vi "AIT 429 Parameter Page.vi"(8 "error in (no error)":errorcluster, 11 "Node Ptr":T3 format="%.0x") -> (0 "error out":errorcluster)   [LabVIEW 2011, in "AIT 429 Custom Device.lvlib"]
uses:
  AIT 429 Custom Device.lvlib
  <vilib>/NI Veristand/Custom Device API/Custom Device Item Ref.ctl
  Controls and Global/Start Bit.ctl
  Controls and Global/Number of Bits.ctl
  Controls and Global/Global.vi
  <vilib>/NI Veristand/Custom Device API/Get Item Property (U32).vi
  <vilib>/NI Veristand/Custom Device API/Get Item Property (Boolean).vi
  <vilib>/NI Veristand/Custom Device API/Get Item Property (Double).vi
  <vilib>/NI Veristand/Custom Device API/Get Item Property (I32).vi
  <vilib>/NI Veristand/Custom Device API/Set Item Property (I32).vi
  <vilib>/NI Veristand/Custom Device API/Set Item Property (Boolean).vi
  <vilib>/NI Veristand/Custom Device API/Set Item Property (Double).vi
  <vilib>/NI Veristand/Custom Device API/Custom Device API.lvlib
panel:
  out "TiggerDValChange":bool
  in  "Scale Offset":dbl format="%#_6f"
  in  "Scale Factor":dbl format="%#_6f"
  in  "Signed?":bool
  out "Default Value":dbl
  in  "Number of Bits":T1=1 min=1 max=32
  in  "Start Bit":T2=1
  in  "Header":cluster{"Section Name":string}={"Section Name"="AIT 429 Parameter"}
  in  "Description":string
  in  "Name":string
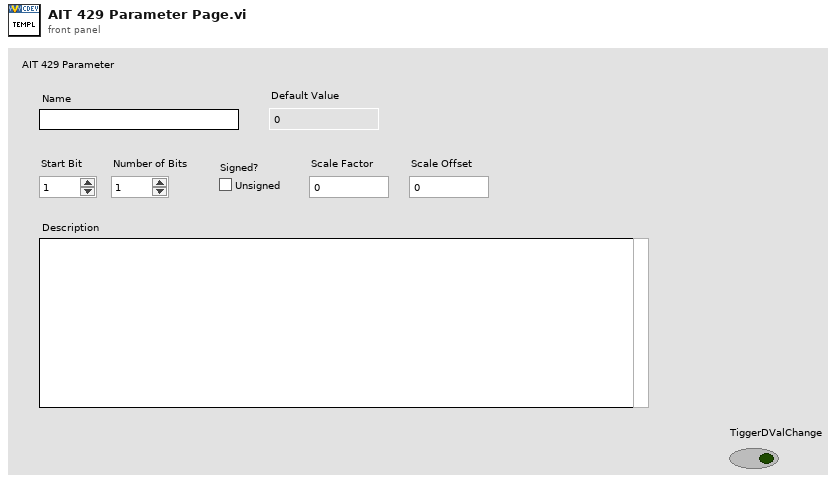
[diagram p1: front panel]
types:
  T1 = typedef "AIT 429 Custom Device.lvlib/Number of Bits.ctl" = i32
  T2 = typedef "AIT 429 Custom Device.lvlib/Start Bit.ctl" = i32
  T3 = typedef "Custom Device API.lvlib/Custom Device Item Ref.ctl" = u64
  T4 = typedef "Custom Device API.lvlib/Custom Device Item Info.ctl" = cluster{"Name":string, "Is Channel":bool, "GUID":string}
  T5 = typedef "Custom Device API.lvlib/Custom Device Channel.ctl" = cluster{"Type":T6, "Units":string, "Default Value":dbl, "Faultable":bool, "Scalable":bool}
  T6 = typedef "Custom Device API.lvlib/Custom Device Channel Type.ctl" = enum16{"Input", "Output"}
  T7 = typedef "Custom Device API.lvlib/Custom Device Commands.ctl" = enum16{"Default", "Item renamed", "Shutdown", "Dynamic button pressed"}
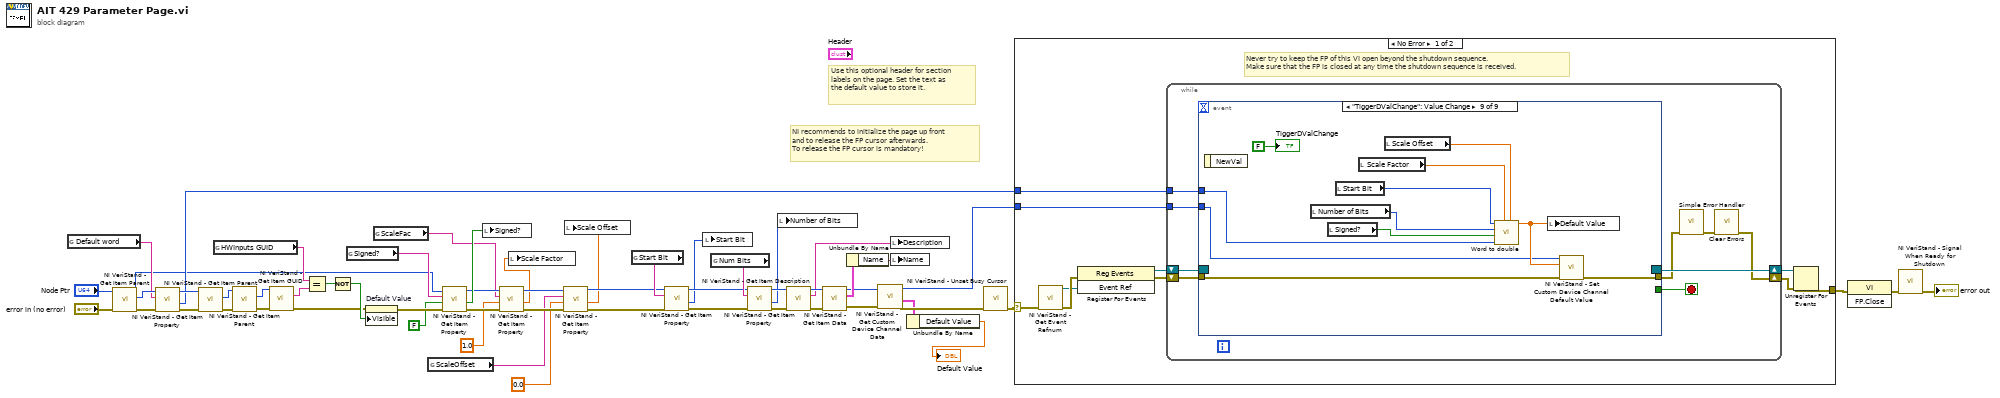
[diagram p0: block diagram]
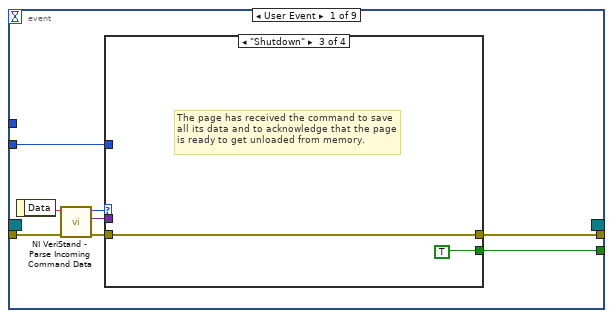
[diagram p2: hidden frame]
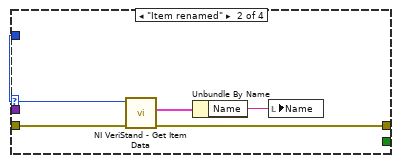
[diagram p4: hidden frame]
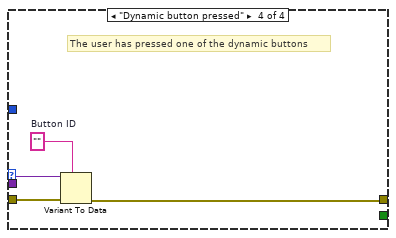
[diagram p5: hidden frame]
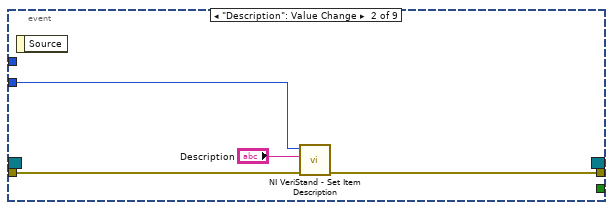
[diagram p6: hidden frame]
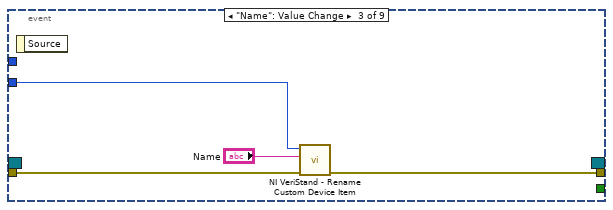
[diagram p7: hidden frame]
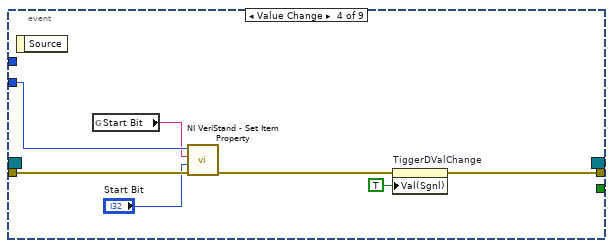
[diagram p8: hidden frame]
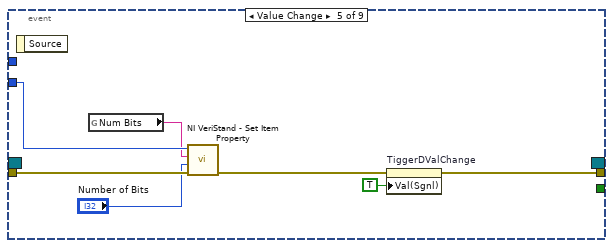
[diagram p9: hidden frame]
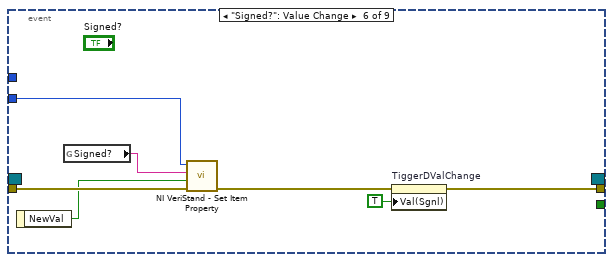
[diagram p10: hidden frame]
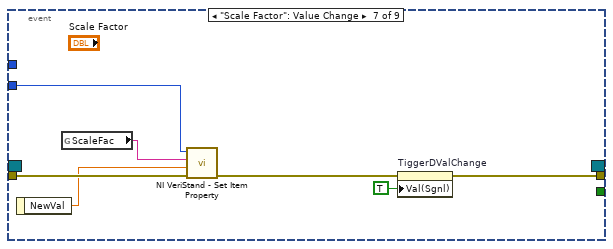
[diagram p11: hidden frame]
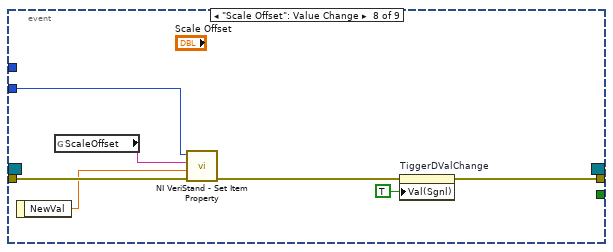
[diagram p12: hidden frame]
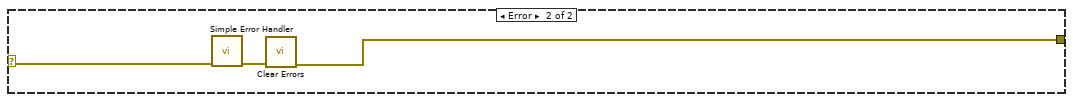
[diagram p13: hidden frame]
diagram:
  # "Use this optional header for section labels on the page. Set the text as the default value to store it."
  # "NI recommends to initialize the page up front\nand to release the FP cursor afterwards.\nTo release the FP cursor is mandatory!"
  n1 = global read "Global.vi" "Default word"() -> (w21:string)
  n2 = call <vilib>:"NI VeriStand - Get Item Parent.vi"("error in (no error)"="error in (no error)", "Item Ref in"="Node Ptr") -> ("error out"=w24:errorcluster, "Parent Ref"=w23:T3, "Item Ref out"=w3:T3)  [unwired: 6 in, 1 out]
  n3 = call-poly <vilib>:"NI VeriStand - Get Item Property.vi"("error in (no error)"=w24, "Property Name"=w21, "Item Ref in"=w23) -> ("error out"=w20:errorcluster, "Value"=w19:u32, "Item Ref out"=w22:T3)  [unwired: 5 in, 1 out]
  n4 = call <vilib>:"NI VeriStand - Get Item Parent.vi"("error in (no error)"=w20, "Item Ref in"=w22) -> ("error out"=w27:errorcluster, "Parent Ref"=w26:T3)  [unwired: 6 in, 2 out]
  n5 = global read "Global.vi" "HWInputs GUID"() -> (w35:string)
  n6 = call <vilib>:"NI VeriStand - Get Item Parent.vi"("error in (no error)"=w27, "Item Ref in"=w26) -> ("error out"=w38:errorcluster, "Parent Ref"=w37:T3)  [unwired: 6 in, 2 out]
  n7 = call <vilib>:"NI VeriStand - Get Item GUID.vi"("error in (no error)"=w38, "Item Ref in"=w37) -> ("error out"=w18:errorcluster, "GUID"=w36:string)  [unwired: 7 in, 1 out]
  n8 = Equal?(x=w35, y=w36) -> (x = y?=w29:bool)
  n9 = Not(x=w29) -> (.not. x?=w28:bool)
  n10 = global read "Global.vi" "Signed?"() -> (w16:string)
  n11 = property on="Default Value" class="DigNum (strict)"(error in=w18, "Visible"=w28) -> (error out=w17:errorcluster)  [unwired: 1 in, 1 out]
  n12 = global read "Global.vi" "ScaleFac"() -> (w11:string)
  n13 = global read "Global.vi" "ScaleOffset"() -> (w5:string)
  n14 = call-poly <vilib>:"NI VeriStand - Get Item Property.vi"("error in (no error)"=w17, "Default Value"=FALSE, "Property Name"=w16, "Item Ref in"=w3) -> ("error out"=w13:errorcluster, "Value"=w14:bool, "Item Ref out"=w12:T3)  [unwired: 4 in, 1 out]
  n15 = local write "Signed?"(w14) -> ()
  n16 = call-poly <vilib>:"NI VeriStand - Get Item Property.vi"("error in (no error)"=w13, "Default Value"=1.0 ("Scale Factor"), "Property Name"=w11, "Item Ref in"=w12) -> ("error out"=w9:errorcluster, "Value"=w1:dbl, "Item Ref out"=w8:T3)  [unwired: 4 in, 1 out]
  n17 = local write "Scale Factor"(w1) -> ()
  n18 = call-poly <vilib>:"NI VeriStand - Get Item Property.vi"("error in (no error)"=w9, "Default Value"=0.0 ("Scale Factor"), "Property Name"=w5, "Item Ref in"=w8) -> ("error out"=w7:errorcluster, "Value"=w2:dbl, "Item Ref out"=w6:T3)  [unwired: 4 in, 1 out]
  n19 = local write "Scale Offset"(w2) -> ()
  n20 = global read "Global.vi" "Start Bit"() -> (w45:string)
  n21 = call-poly <vilib>:"NI VeriStand - Get Item Property.vi"("error in (no error)"=w7, "Property Name"=w45, "Item Ref in"=w6) -> ("error out"=w43:errorcluster, "Value"=w42:i32, "Item Ref out"=w44:T3)  [unwired: 5 in, 1 out]
  n22 = local write "Start Bit"(w42) -> ()
  n23 = global read "Global.vi" "Num Bits"() -> (w48:string)
  n24 = call-poly <vilib>:"NI VeriStand - Get Item Property.vi"("error in (no error)"=w43, "Property Name"=w48, "Item Ref in"=w44) -> ("error out"=w46:errorcluster, "Value"=w41:i32, "Item Ref out"=w47:T3)  [unwired: 5 in, 1 out]
  n25 = local write "Number of Bits"(w41) -> ()
  n26 = call <vilib>:"NI VeriStand - Get Item Description.vi"("error in (no error)"=w46, "Item Ref in"=w47) -> ("error out"=w51:errorcluster, "Description"=w52:string, "Item Ref out"=w53:T3)  [unwired: 7 out]
  n27 = call <vilib>:"NI VeriStand - Get Item Data.vi"("error in (no error)"=w51, "Item Ref in"=w53) -> ("error out"=w34:errorcluster, "Item Info"=w50:T4, "Item Ref out"=w33:T3)  [unwired: 7 out]
  n28 = Unbundle By Name(w50) -> ("Name"=w49:string)
  n29 = call <vilib>:"NI VeriStand - Get Custom Device Channel Data.vi"("error in (no error)"=w34, "Channel Ref in"=w33) -> ("error out"=w31:errorcluster, "Channel"=w30:T5, "Channel Ref out"=w32:T3)  [unwired: 4 in, 3 out]
  n30 = local write "Description"(w52) -> ()
  n31 = local write "Name"(w49) -> ()
  n32 = Unbundle By Name(w30) -> ("Default Value"=→"Default Value":dbl)
  n33 = call <vilib>:"NI VeriStand - Unset Busy Cursor.vi"("error in (no error)"=w31) -> ("error out"=w54:errorcluster)  [unwired: 10 out]
  n34 = case shown="No Error" w54 {
    selector: w54 -> [w59 w153]
    tunnel: [w64 w151] -> w57
    tunnel: w32 -> [w60 _]
    tunnel: w19 -> [w58 _]
    frame No Error {
      # "Never try to keep the FP of this VI open beyond the shutdown sequence.\nMake sure that the FP is closed at any time the shutdown sequence is received."
      n35 = call <vilib>:"NI VeriStand - Get Event Refnum.vi"("error in (no error)"=w59) -> ("error out"=w67:errorcluster, "Event Ref"=w63:refnum<user-event>)  [unwired: 9 out]
      n36 = register-events(error in=w67, w63) -> (reference out=w61:refnum<event-registration>, error out=w62:errorcluster)  [unwired: 1 in]
      n37 = while {
        tunnel: w60 -> [w72]
        shift-right: [w69] -> w65
        shift-left: w62 -> [w75]
        shift-right: [w76] -> w66
        shift-left: w61 -> [w74]
        tunnel: w58 -> [w68]
        stop <- w73 stop-if-true
        n38 = event shown="[8] \"TiggerDValChange\": Value Change" {
          selector: w74 -> [_ _ _ _ _ _ _ _ _]
          dyn-events: [_ _ _ _ _ _ _ _ _] -> w76
          timeout: _ -> [_ _ _ _ _ _ _ _ _]
          tunnel: w75 -> [w84 w99 w103 w111 w118 w125 w132 w139 w150]
          tunnel: [w80 _ _ _ _ _ _ _ _] -> w73
          tunnel: [w79 w98 w102 w106 w112 w119 w126 w133 w149] -> w71
          tunnel: w72 -> [w78 w100 w104 w110 w117 w124 w131 w138 w147]
          tunnel: w68 -> [_ _ _ _ _ _ _ _ w146]
          event User Event {
            n39 = event-data() -> ("Data"=w83:string)  [unwired: 1 out]
            n40 = call <vilib>:"NI VeriStand - Parse Incoming Command Data.vi"("error in (no error)"=w84, "Incoming data"=w83) -> ("error out"=w82:errorcluster, "Outgoing data"=w77:variant, "Action"=w81:T7)  [unwired: 7 out]
            n41 = case shown="\"Shutdown\"" w81 {
              tunnel: w82 -> [w85 w90 w91 w96]
              tunnel: [_ _ TRUE _] -> w80
              tunnel: [w85 w87 w91 w93] -> w79
              tunnel: w78 -> [_ w89 _ _]
              tunnel: w77 -> [_ _ _ w95]
              frame "Default", Default {
              }
              frame "Item renamed" {
                n42 = call <vilib>:"NI VeriStand - Get Item Data.vi"("error in (no error)"=w90, "Item Ref in"=w89) -> ("error out"=w87:errorcluster, "Item Info"=w88:T4)  [unwired: 8 out]
                n43 = Unbundle By Name(w88) -> ("Name"=w86:string)
                n44 = local write "Name"(w86) -> ()
              }
              frame "Shutdown" {
                # "The page has received the command to save all its data and to acknowledge that the page is ready to get unloaded from memory."
              }
              frame "Dynamic button pressed" {
                w94 = ""  # Button ID
                # "The user has pressed one of the dynamic buttons"
                n45 = Variant To Data(error in=w96, type=w94, Variant=w95) -> (error out=w93:errorcluster)  [unwired: 1 out]
              }
            }
          }
          event "Description": Value Change {
            n46 = event-data() -> ()  [unwired: 2 out]
            n47 = call <vilib>:"NI VeriStand - Set Item Description.vi"("error in (no error)"=w99, "Description"="Description", "Item Ref in"=w100) -> ("error out"=w98:errorcluster)  [unwired: 8 out]
          }
          event "Name": Value Change {
            n48 = event-data() -> ()  [unwired: 2 out]
            n49 = call <vilib>:"NI VeriStand - Rename Custom Device Item.vi"("error in (no error)"=w103, "New Name"="Name", "Item Ref in"=w104) -> ("error out"=w102:errorcluster)  [unwired: 6 in, 2 out]
          }
          event Value Change {
            n50 = event-data() -> ()  [unwired: 2 out]
            n51 = global read "Global.vi" "Start Bit"() -> (w109:string)
            n52 = call-poly <vilib>:"NI VeriStand - Set Item Property.vi"("error in (no error)"=w111, "Value"="Start Bit", "Property Name"=w109, "Item Ref in"=w110) -> ("error out"=w107:errorcluster)  [unwired: 5 in, 2 out]
            n53 = property on="TiggerDValChange" class="Bool (strict)"(error in=w107, "Val(Sgnl)"=TRUE ("Value (Signaling)")) -> (error out=w106:errorcluster)  [unwired: 1 in, 1 out]
          }
          event Value Change {
            n54 = event-data() -> ()  [unwired: 2 out]
            n55 = global read "Global.vi" "Num Bits"() -> (w116:string)
            n56 = call-poly <vilib>:"NI VeriStand - Set Item Property.vi"("error in (no error)"=w118, "Value"="Number of Bits", "Property Name"=w116, "Item Ref in"=w117) -> ("error out"=w113:errorcluster)  [unwired: 5 in, 2 out]
            n57 = property on="TiggerDValChange" class="Bool (strict)"(error in=w113, "Val(Sgnl)"=TRUE ("Value (Signaling)")) -> (error out=w112:errorcluster)  [unwired: 1 in, 1 out]
          }
          event "Signed?": Value Change {
            n58 = event-data() -> ("NewVal"=w122:bool)  [unwired: 1 out]
            n59 = global read "Global.vi" "Signed?"() -> (w123:string)
            n60 = call-poly <vilib>:"NI VeriStand - Set Item Property.vi"("error in (no error)"=w125, "Value"=w122, "Property Name"=w123, "Item Ref in"=w124) -> ("error out"=w120:errorcluster)  [unwired: 5 in, 2 out]
            n61 = property on="TiggerDValChange" class="Bool (strict)"(error in=w120, "Val(Sgnl)"=TRUE ("Value (Signaling)")) -> (error out=w119:errorcluster)  [unwired: 1 in, 1 out]
          }
          event "Scale Factor": Value Change {
            n62 = event-data() -> ("NewVal"=w129:dbl)  [unwired: 1 out]
            n63 = global read "Global.vi" "ScaleFac"() -> (w130:string)
            n64 = call-poly <vilib>:"NI VeriStand - Set Item Property.vi"("error in (no error)"=w132, "Value"=w129, "Property Name"=w130, "Item Ref in"=w131) -> ("error out"=w127:errorcluster)  [unwired: 5 in, 2 out]
            n65 = property on="TiggerDValChange" class="Bool (strict)"(error in=w127, "Val(Sgnl)"=TRUE ("Value (Signaling)")) -> (error out=w126:errorcluster)  [unwired: 1 in, 1 out]
          }
          event "Scale Offset": Value Change {
            n66 = event-data() -> ("NewVal"=w136:dbl)  [unwired: 1 out]
            n67 = global read "Global.vi" "ScaleOffset"() -> (w137:string)
            n68 = call-poly <vilib>:"NI VeriStand - Set Item Property.vi"("error in (no error)"=w139, "Value"=w136, "Property Name"=w137, "Item Ref in"=w138) -> ("error out"=w134:errorcluster)  [unwired: 5 in, 2 out]
            n69 = property on="TiggerDValChange" class="Bool (strict)"(error in=w134, "Val(Sgnl)"=TRUE ("Value (Signaling)")) -> (error out=w133:errorcluster)  [unwired: 1 in, 1 out]
          }
          event "TiggerDValChange": Value Change {
            n70 = event-data() -> ()  [unwired: 2 out]
            n71 = local read "Number of Bits"() -> (w144:T1)
            n72 = local read "Signed?"() -> (w145:bool)
            n73 = local read "Start Bit"() -> (w143:T2)
            n74 = local read "Scale Factor"() -> (w142:dbl)
            n75 = local read "Scale Offset"() -> (w141:dbl)
            n76 = call "Word to double.vi"("ScaleOffset (0)"=w141, "ScaleFac (1)"=w142, "word"=w146, "Signed? (F)"=w145, "Number of Bits"=w144, "Start Bit"=w143) -> ("Double"=w148:dbl)  [unwired: 5 in]
            n77 = local write "Default Value"(w148) -> ()
            n78 = call <vilib>:"NI VeriStand - Set Custom Device Channel Default Value.vi"("error in (no error)"=w150, "Default Value"=w148, "Channel Ref in"=w147) -> ("error out"=w149:errorcluster)  [unwired: 7 in, 1 out]
            "TiggerDValChange" <- FALSE
          }
        }
        n79 = call <vilib>:"Simple Error Handler.vi"("error in (no error)"=w71) -> ("error out"=w70:errorcluster)  [unwired: 1 in, 7 out]
        n80 = call <vilib>:"Clear Errors.vi"("error in (no error)"=w70) -> ("error out"=w69:errorcluster)  [unwired: 6 out]
      }
      n81 = Unregister For Events(event registration refnum=w66, error in=w65) -> (error out=w64:errorcluster)
    }
    frame Error {
      n82 = call <vilib>:"Simple Error Handler.vi"("error in (no error)"=w153) -> ("error out"=w152:errorcluster)  [unwired: 1 in, 7 out]
      n83 = call <vilib>:"Clear Errors.vi"("error in (no error)"=w152) -> ("error out"=w151:errorcluster)  [unwired: 6 out]
    }
  }
  n84 = invoke class="VI" method="FP.Close"(error in=w57) -> (error out=w56:errorcluster)  [unwired: 2 in, 2 out]
  n85 = call <vilib>:"NI VeriStand - Signal When Ready for Shutdown.vi"("error in (no error)"=w56) -> ("error out"=→"error out":errorcluster)  [unwired: 10 out]
